vi "alarmclock.vi"() -> ()   [LabVIEW 2017]
panel:
  out "Date":string
  in  "x 3":dbl
  in  "Hour":dbl
  in  "Mintues":dbl
  out "Alarm":bool
  in  "variabe 2":bool
  in  "variabe":bool
  in  "?":bool
  out "Time":string
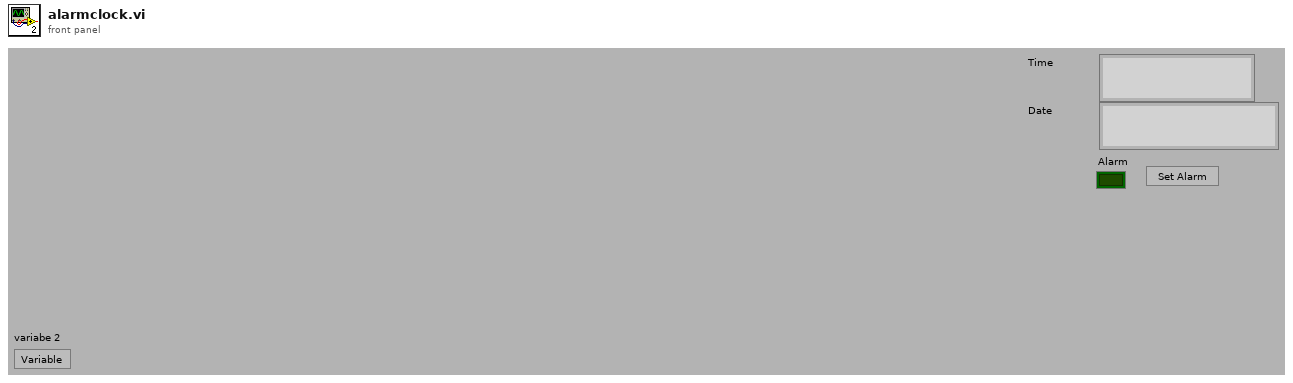
[diagram p1: front panel]
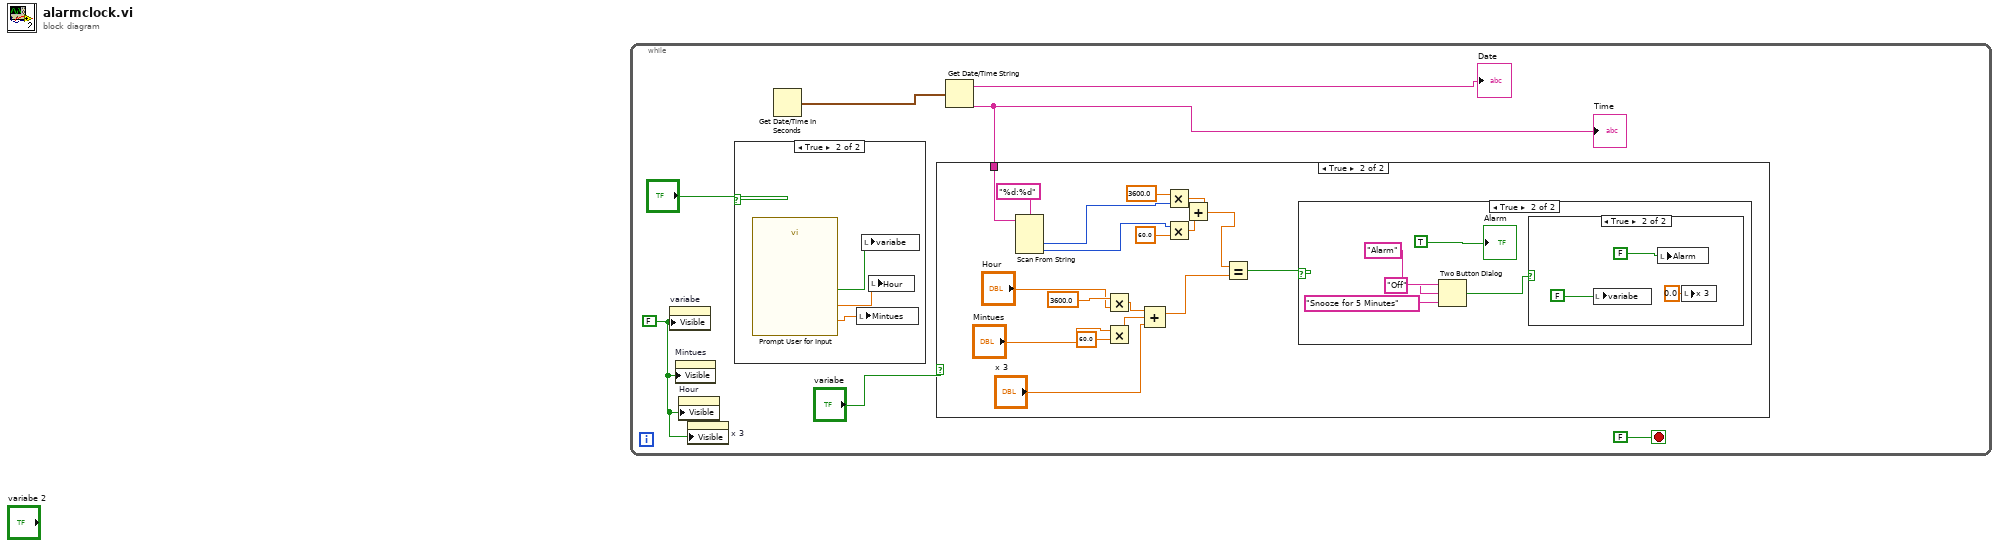
[diagram p0: block diagram]
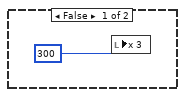
[diagram p4: hidden frame]
diagram:
  n1 = while {
    stop <- FALSE stop-if-true
    w2 = FALSE ("Visible")
    n2 = property on="variabe" class="Bool (strict)"("Visible"=w2) -> ()  [unwired: 2 in, 2 out]
    n3 = property on="Mintues" class="DigNum (strict)"("Visible"=w2) -> ()  [unwired: 2 in, 2 out]
    n4 = property on="Hour" class="DigNum (strict)"("Visible"=w2) -> ()  [unwired: 2 in, 2 out]
    n5 = property on="x 3" class="DigNum (strict)"("Visible"=w2) -> ()  [unwired: 2 in, 2 out]
    n6 = case shown="True" "?" {
      frame False {
      }
      frame True {
        n7 = call "Prompt User for Input"() -> ("Minute"=w35:dbl, "Hour"=w36:dbl, "OK"=w37:bool)  [unwired: 16 in, 1 out]
        n8 = local write "Mintues"(w35) -> ()
        n9 = local write "variabe"(w37) -> ()
        n10 = local write "Hour"(w36) -> ()
      }
    }
    n11 = Get Date/Time In Seconds() -> (seconds since 1Jan1904=w4:timestamp)
    n12 = Get Date/Time String(seconds (now)=w4) -> (date string=→"Date":string, time string=w3:string)  [unwired: 2 in]
    "Time" <- w3
    n13 = case shown="True" "variabe" {
      tunnel: w3 -> [_ w11]
      frame False {
      }
      frame True {
        n14 = Scan From String(format string="%d:%d", input string=w11) -> (output 1=w10:i32, output 2=w9:i32)  [unwired: 4 in, 3 out]
        n15 = Multiply(x=3600.0, y="Hour") -> (x*y=w23:dbl)
        n16 = Multiply(x="Mintues", y=60.0) -> (x*y=w22:dbl)
        n17 = Compound Arithmetic op=ADD(w23, w22, "x 3") -> (w18:dbl)
        n18 = Multiply(x=3600.0, y=w10) -> (x*y=w15:dbl)
        n19 = Multiply(x=w9, y=60.0) -> (x*y=w14:dbl)
        n20 = Add(x=w15, y=w14) -> (x+y=w13:dbl)
        n21 = Equal?(x=w13, y=w18) -> (x = y?=w21:bool)
        n22 = case shown="True" w21 {
          frame False {
          }
          frame True {
            n23 = Two Button Dialog(message="Alarm", 1:"Snooze for 5 Minutes" ("F button name (\"Cancel\")"), 2:"Off" ("T button name (\"OK\")")) -> (T button?=w27:bool)
            n24 = case shown="True" w27 {
              frame False {
                n25 = local write "x 3"(300) -> ()
              }
              frame True {
                n26 = local write "variabe"(FALSE ("variabe")) -> ()
                n27 = local write "Alarm"(FALSE ("Alarm")) -> ()
                n28 = local write "x 3"(0.0 ("x 3")) -> ()
              }
            }
            "Alarm" <- TRUE ("Boolean")
          }
        }
      }
    }
  }
